vi "Main.vi"() -> ()   [LabVIEW 2021]
uses:
  <vilib>/Instr/_visa.llb/VISA Configure Serial Port (Instr).vi
panel:
  out "read buffer":string
  out "Waveform Chart":cluster{"omega":sgl, "current":sgl}(graph)
  out "error out":errorcluster
  out "Cluster":cluster{"omega":sgl, "current":sgl}
  in  "VISA resource name":refnum<visa-resource-name>
  in  "stop":bool
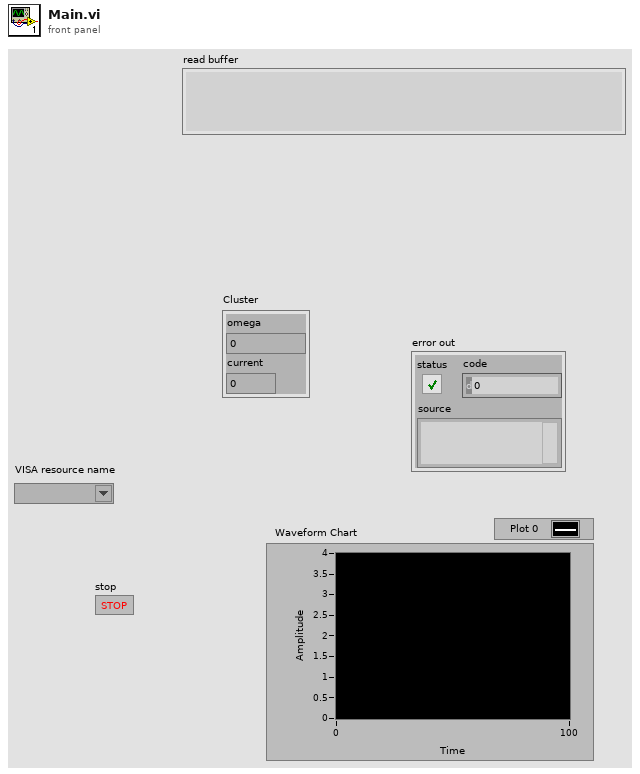
[diagram p1: front panel]
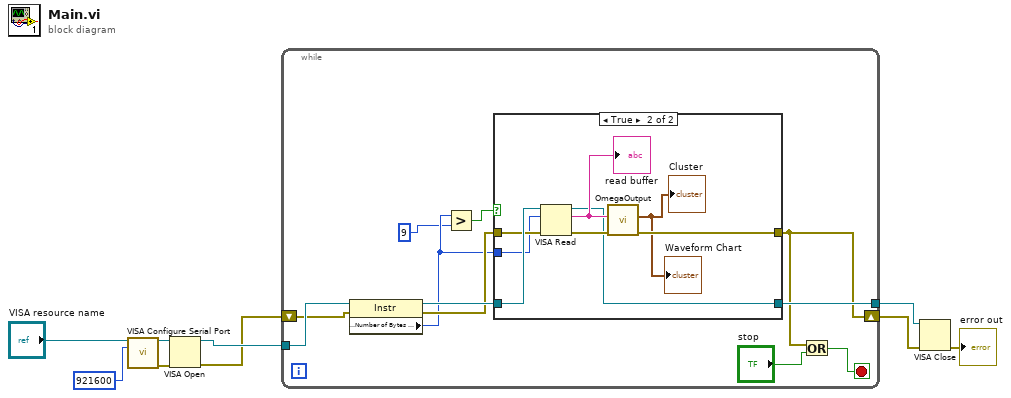
[diagram p0: block diagram]
diagram:
  n1 = call-poly "VISA Configure Serial Port"("VISA resource name"="VISA resource name", "baud rate (9600)"=u32 921600) -> ("VISA resource name out"=w7:refnum<visa-resource-name>, "error out"=w5:errorcluster)  [unwired: 12 in]
  n2 = VISA Open(error in (no error)=w5, VISA resource name=w7) -> (VISA resource name=w6:refnum<visa-resource-name>, error out=w4:errorcluster)  [unwired: 3 in]
  n3 = while {
    tunnel: w6 -> [w20]
    shift-right: [w13] -> w3
    shift-left: w4 -> [w18]
    tunnel: [w16] -> w2
    stop <- w14 stop-if-true
    n4 = property class="Instr"(reference=w20, error in=w18) -> (reference out=w19:refnum<visa-resource-name>, error out=w17:errorcluster, "Serial Settings:Number of Bytes at Serial Port"=w11:u32)
    n5 = Greater?(x=w11, y=u32 9 ("x")) -> (0:w12:bool)
    n6 = case shown="True" w12 {
      tunnel: w19 -> [w21 w30]
      tunnel: w17 -> [w22 w28]
      tunnel: [w22 w26] -> w13
      tunnel: [w21 w25] -> w16
      tunnel: w11 -> [_ w23]
      frame False {
      }
      frame True {
        n7 = VISA Read(VISA resource name=w30, byte count=w23, error in (no error)=w28) -> (VISA resource name out=w25:refnum<visa-resource-name>, read buffer=w29:string, error out=w27:errorcluster)  [unwired: 1 out]
        "read buffer" <- w29
        n8 = call "OmegaOutput.vi"("error in (no error)"=w27, "String"=w29) -> ("error out"=w26:errorcluster, "Cluster"=→"Cluster" →"Waveform Chart":cluster{"omega":sgl, "current":sgl})  [unwired: 8 in]
      }
    }
    n9 = Or(x=w13, y="stop") -> (x .or. y?=w14:bool)
  }
  n10 = VISA Close(VISA resource name=w2, error in (no error)=w3) -> (error out=→"error out":errorcluster)
